vi "Measurement Logic.vi"() -> ()   [LabVIEW 2021, in "Advanced Data Structure Exchange.lvlib"]
uses:
  Advanced Data Structure Exchange.lvlib
  Measurement Configuration.ctl
  Measurement Results.ctl
  <vilib>/MeasurementLink/MeasurementLink Measurement Server/Measure Call Context/Measure Call Context.lvclass
  Cluster In.ctl
  2dd92f02-7c25-4401-8305-04303adf7e71.vi
  944e2848-8240-4935-bcfe-6d4ed07f3af2.vi
  e8695424-5121-4886-9511-2a80180f6bad.vi
  70be038f-b641-41bc-a58d-b8dc7123d6da.vi
  <vilib>/JDP Science/JSONtext/JSON text to Variant.vi
  <vilib>/JDP Science/JSONtext/Variant to JSON Text.vi
  <vilib>/JDP Science/JSONtext/LVClass Serializer/JSONtext LVClass Serializer.lvclass
panel:
  out "measure call context out":refnum<class "Measure Call Context.lvclass">
  in  "measure call context in":refnum<class "Measure Call Context.lvclass">
  out "measurement results":T1
  in  "measurement configuration":T2
  out "error out":errorcluster
  in  "error in":errorcluster
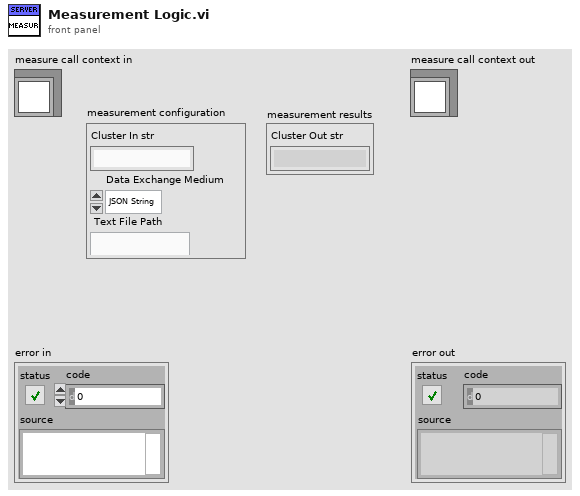
[diagram p1: front panel]
types:
  T1 = typedef "Advanced Data Structure Exchange.lvlib/Measurement Results.ctl" = cluster{"Cluster Out str":string}
  T2 = typedef "Advanced Data Structure Exchange.lvlib/Measurement Configuration.ctl" = cluster{"Cluster In str":string, "Data Exchange Medium":enum32{"JSON String", "Text File"}, " Text File Path":string}
  T3 = typedef "Advanced Data Structure Exchange.lvlib/Cluster In.ctl" = cluster{"Numeric":dbl, "Bool 2D Array":bool[][], "String 2D Array":string[][], "Text Ring":u16, "Cluster":cluster{"Num Array":dbl[], "Bool Array":bool[]}, "Time Stamp":timestamp, "Enum":enum16{"DC Voltage", "DC Current"}, "DAQmx Physical Channel":tag, "Combo Box":string, "Cluster Array":cluster{"Numeric 2D Array":dbl[][], "Cluster Nest":cluster{"String Array":string[], "Bool Array":bool[], "Cluster in Cluster":cluster{"Numeric":dbl, "Boolean":bool, "String":string}}}[]}
  T4 = enum16{"open", "replace", "create", "open or create", "replace or create", "replace or create with confirmation"}
  T5 = cluster{"Numeric 2D Array":dbl[][], "Cluster Nest":cluster{"String Array":string[], "Bool Array":bool[], "Cluster in Cluster":cluster{"Numeric":dbl, "Boolean":bool, "String":string}}}[]
  T6 = cluster{"Numeric 2D Array":dbl[][], "Cluster Nest":cluster{"String Array":string[], "Bool Array":bool[], "Cluster in Cluster":cluster{"Numeric":dbl, "Boolean":bool, "String":string}}}
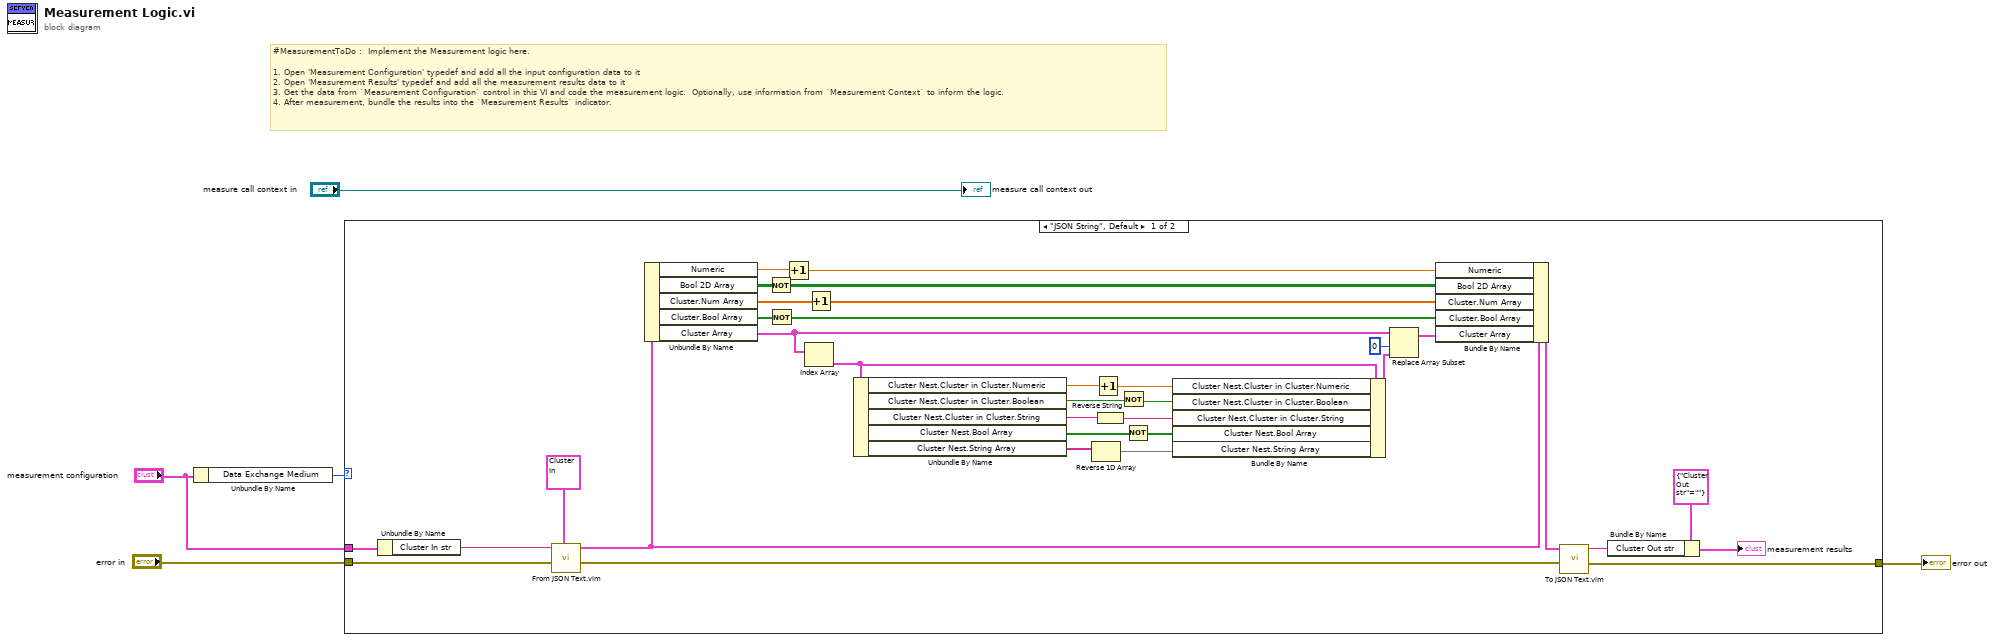
[diagram p0: block diagram]
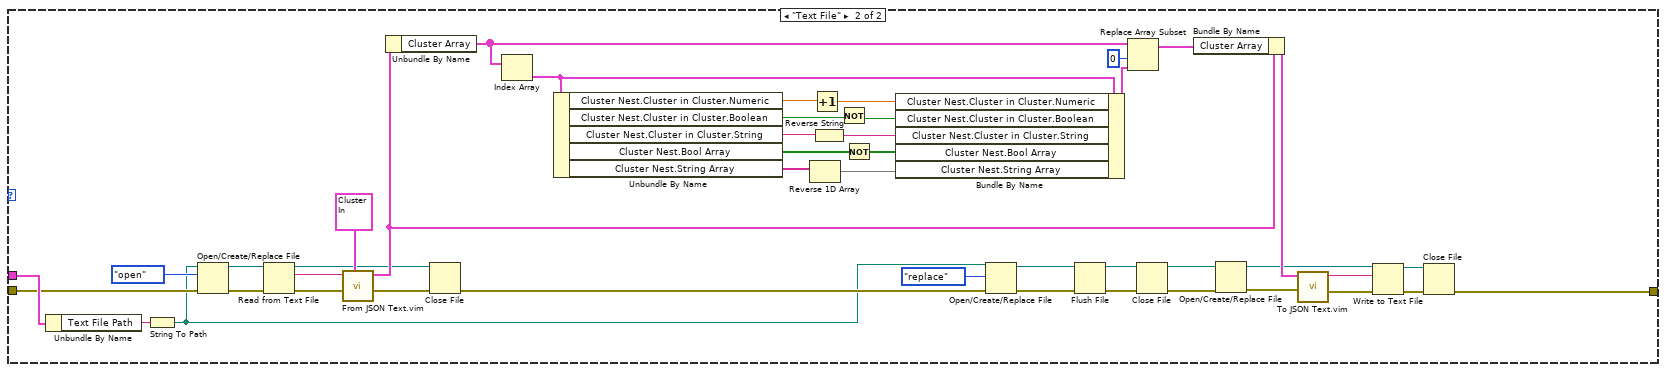
[diagram p2: hidden frame]
diagram:
  # "#MeasurementToDo :  Implement the Measurement logic here.\n\n1. Open 'Measurement Configuration' typedef and add all the input configuration data to it\n2. Open 'Measurement Results' typedef and add all the measurement results data to it\n3. Get the data from `Measurement Configuration` control in this VI and code the measurement logic.  Optionally, use information from `Measurement Context` to inform the logic.\n4. After measurement, bundle the results into the `Measurement Results` indicator."
  n1 = Unbundle By Name("measurement configuration") -> ("Data Exchange Medium"=w1:enum32{"JSON String", "Text File"})
  n2 = case shown="\"JSON String\", Default" w1 {
    tunnel: "error in" -> [w37 w61]
    tunnel: [w17 w46] -> w3
    tunnel: "measurement configuration" -> [w10 w66]
    frame "JSON String", Default {
      n3 = Unbundle By Name(w10) -> ("Cluster In str"=w38:string)
      n4 = call "From JSON Text.vim"("Data Type and Default Value"=T3 {"Numeric"=0.0, "Bool 2D Array"=[], "String 2D Array"=[], "Text Ring"=0, "Cluster"={"Num Array"=[], "Bool Array"=[]}, "Time Stamp"=timestamp(0 s since 1904-01-01), "Enum"=enum."DC Voltage", "DAQmx Physical Channel"="", "Combo Box"="", "Cluster Array"=[]} ("Cluster In"), "error in (no error)"=w37, "JSON"=w38) -> ("error out"=w9:errorcluster, "Data out"=w15:T3)  [unwired: 7 in]
      n5 = Unbundle By Name(w15) -> ("Numeric"=w33:dbl, "Bool 2D Array"=w32:bool[][], "Cluster.Num Array"=w34:dbl[], "Cluster.Bool Array"=w31:bool[], "Cluster Array"=w19:T5)
      n6 = Not(x=w32) -> (.not. x?=w29:bool[][])
      n7 = Not(x=w31) -> (.not. x?=w27:bool[])
      n8 = Increment(x=w33) -> (x+1=w30:dbl)
      n9 = Index Array(array=w19) -> (element=w23:T6)  [unwired: 1 in]
      n10 = Increment(x=w34) -> (x+1=w28:dbl[])
      n11 = Unbundle By Name(w23) -> ("Cluster Nest.Cluster in Cluster.Numeric"=w25:dbl, "Cluster Nest.Cluster in Cluster.Boolean"=w24:bool, "Cluster Nest.Cluster in Cluster.String"=w26:string, "Cluster Nest.Bool Array"=w14:bool[], "Cluster Nest.String Array"=w12:string[])
      n12 = Reverse 1D Array(array=w12) -> (reversed array=w11:string[])
      n13 = Increment(x=w25) -> (x+1=w22:dbl)
      n14 = Reverse String(1:w26) -> (0:w20:string)
      n15 = Not(x=w24) -> (.not. x?=w21:bool)
      n16 = Not(x=w14) -> (.not. x?=w13:bool[])
      n17 = Bundle By Name(cluster=w23, "Cluster Nest.Cluster in Cluster.Numeric"=w22, "Cluster Nest.Cluster in Cluster.Boolean"=w21, "Cluster Nest.Cluster in Cluster.String"=w20, "Cluster Nest.Bool Array"=w13, "Cluster Nest.String Array"=w11) -> (w7:T6)
      n18 = Replace Array Subset(array=w19, new element=w7, index=0) -> (w18:T5)
      n19 = Bundle By Name(cluster=w15, "Numeric"=w30, "Bool 2D Array"=w29, "Cluster.Num Array"=w28, "Cluster.Bool Array"=w27, "Cluster Array"=w18) -> (w36:T3)
      n20 = call "To JSON Text.vim"("error in (no error)"=w9, "Anything"=w36) -> ("error out"=w17:errorcluster, "<JSON>"=w35:string)  [unwired: 8 in]
      n21 = Bundle By Name(cluster=T1 {"Cluster Out str"=""} ("measurement results"), "Cluster Out str"=w35) -> (→"measurement results":T1)
    }
    frame "Text File" {
      n22 = Unbundle By Name(w66) -> ("Text File Path"=w62:string)
      n23 = String To Path(string=w62) -> (path=w43:path)
      n24 = Open/Create/Replace File(file path (use dialog)=w43, error in=w61, operation (0:open)=T4."open") -> (refnum out=w65:refnum<file>, error out=w64:errorcluster)  [unwired: 3 in, 1 out]
      n25 = Read from Text File(file (use dialog)=w65, error in=w64) -> (refnum out=w58:refnum<file>, text=w59:string, error out=w60:errorcluster)  [unwired: 2 in, 1 out]
      n26 = call "From JSON Text.vim"("Data Type and Default Value"=T3 {"Numeric"=0.0, "Bool 2D Array"=[], "String 2D Array"=[], "Text Ring"=0, "Cluster"={"Num Array"=[], "Bool Array"=[]}, "Time Stamp"=timestamp(0 s since 1904-01-01), "Enum"=enum."DC Voltage", "DAQmx Physical Channel"="", "Combo Box"="", "Cluster Array"=[]} ("Cluster In"), "error in (no error)"=w60, "JSON"=w59) -> ("error out"=w57:errorcluster, "Data out"=w71:T3)  [unwired: 7 in]
      n27 = Unbundle By Name(w71) -> ("Cluster Array"=w75:T5)
      n28 = Close File(refnum=w58, error in=w57) -> (error out=w44:errorcluster)  [unwired: 1 out]
      n29 = Index Array(array=w75) -> (element=w79:T6)  [unwired: 1 in]
      n30 = Unbundle By Name(w79) -> ("Cluster Nest.Cluster in Cluster.Numeric"=w81:dbl, "Cluster Nest.Cluster in Cluster.Boolean"=w80:bool, "Cluster Nest.Cluster in Cluster.String"=w82:string, "Cluster Nest.Bool Array"=w70:bool[], "Cluster Nest.String Array"=w68:string[])
      n31 = Reverse 1D Array(array=w68) -> (reversed array=w67:string[])
      n32 = Increment(x=w81) -> (x+1=w78:dbl)
      n33 = Reverse String(1:w82) -> (0:w76:string)
      n34 = Not(x=w80) -> (.not. x?=w77:bool)
      n35 = Not(x=w70) -> (.not. x?=w69:bool[])
      n36 = Bundle By Name(cluster=w79, "Cluster Nest.Cluster in Cluster.Numeric"=w78, "Cluster Nest.Cluster in Cluster.Boolean"=w77, "Cluster Nest.Cluster in Cluster.String"=w76, "Cluster Nest.Bool Array"=w69, "Cluster Nest.String Array"=w67) -> (w73:T6)
      n37 = Open/Create/Replace File(file path (use dialog)=w43, error in=w44, operation (0:open)=T4."replace") -> (refnum out=w54:refnum<file>, error out=w53:errorcluster)  [unwired: 3 in, 1 out]
      n38 = Flush File(refnum=w54, error in=w53) -> (refnum out=w56:refnum<file>, error out=w52:errorcluster)
      n39 = Replace Array Subset(array=w75, new element=w73, index=0) -> (w74:T5)
      n40 = Close File(refnum=w56, error in=w52) -> (path=w55:path, error out=w51:errorcluster)
      n41 = Bundle By Name(cluster=w71, "Cluster Array"=w74) -> (w83:T3)
      n42 = Open/Create/Replace File(file path (use dialog)=w55, error in=w51) -> (refnum out=w41:refnum<file>, error out=w42:errorcluster)  [unwired: 4 in, 1 out]
      n43 = call "To JSON Text.vim"("error in (no error)"=w42, "Anything"=w83) -> ("error out"=w47:errorcluster, "<JSON>"=w48:string)  [unwired: 8 in]
      n44 = Write to Text File(file (use dialog)=w41, text=w48, error in=w47) -> (refnum out=w49:refnum<file>, error out=w45:errorcluster)  [unwired: 1 in, 1 out]
      n45 = Close File(refnum=w49, error in=w45) -> (error out=w46:errorcluster)  [unwired: 1 out]
    }
  }
  "error out" <- w3
  "measure call context out" <- "measure call context in"
